vi "编辑Limit_Line.vi"(9 "引用":refnum<vi>, 11 "Data In":string[](array[string])) -> (1 "Operate":string, 2 "OK？":bool, 3 "Data Out":string[](array[string]))   [LabVIEW 2020]
panel:
  out "Unit 5":string
  out "Unit 4":string
  in  "End Response":dbl
  out "Unit 3":string="Hz"
  in  "End Stimulus":dbl format="%#.0f"
  out "Unit 2":string="Hz"
  in  "复制":bool
  in  "删除":bool
  in  "取消":bool
  in  "确定":bool
  in  "Begin Response":dbl
  in  "Type":u16(ring) items=["OFF", "MAX", "MIN"]
  in  "Begin Stimulus":dbl format="%#.0f"
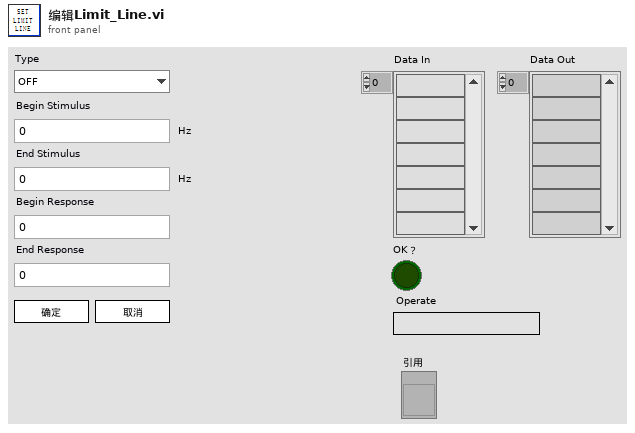
[diagram p1: front panel]
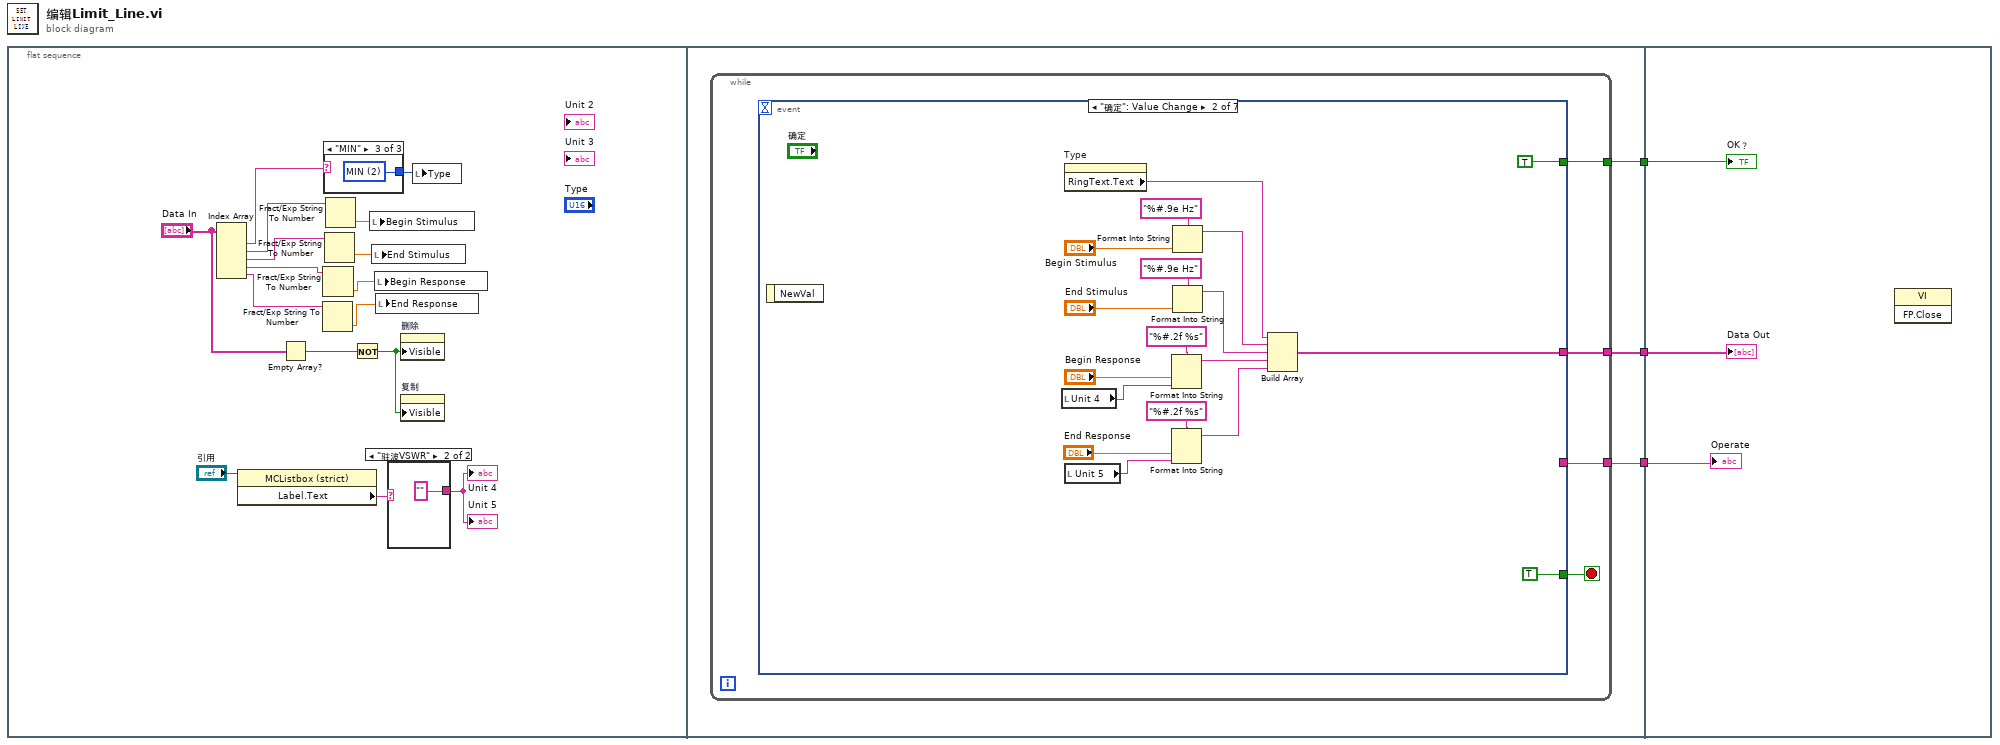
[diagram p0: block diagram]
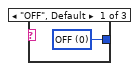
[diagram p2: hidden frame]
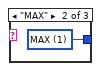
[diagram p3: hidden frame]
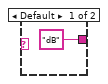
[diagram p4: hidden frame]
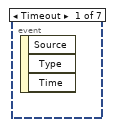
[diagram p5: hidden frame]
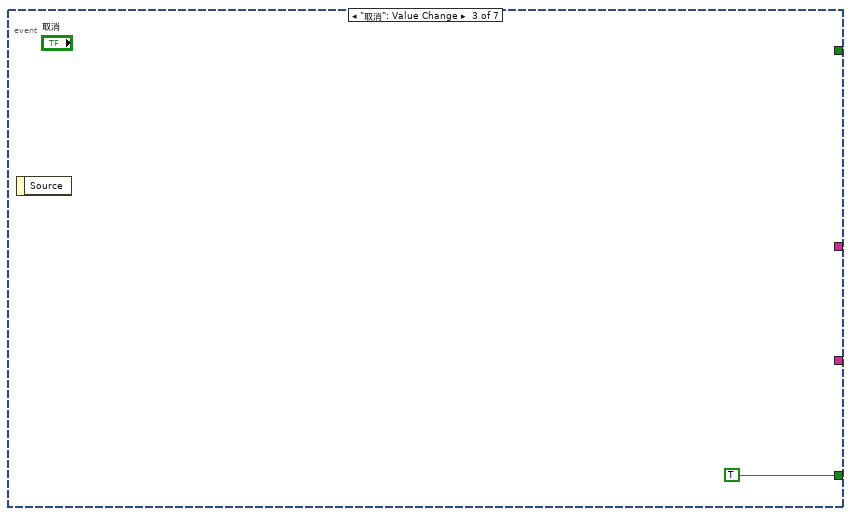
[diagram p6: hidden frame]
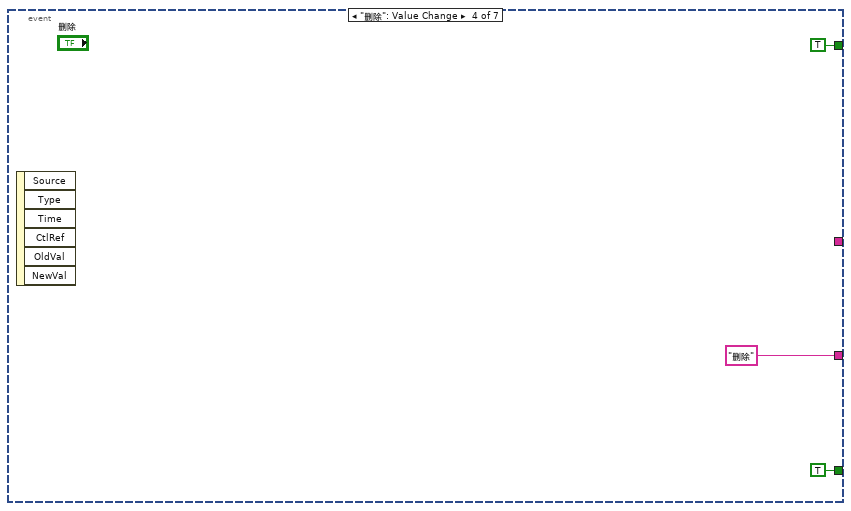
[diagram p7: hidden frame]
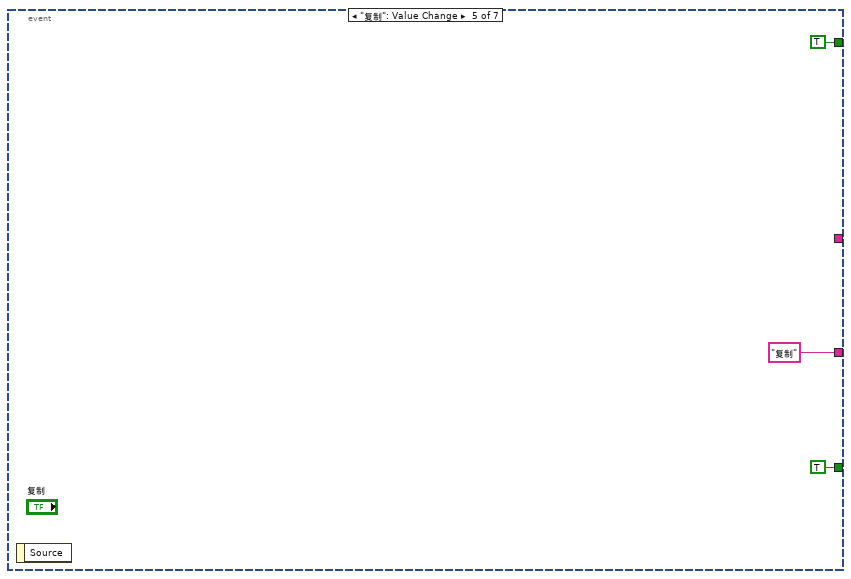
[diagram p8: hidden frame]
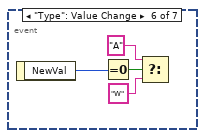
[diagram p9: hidden frame]
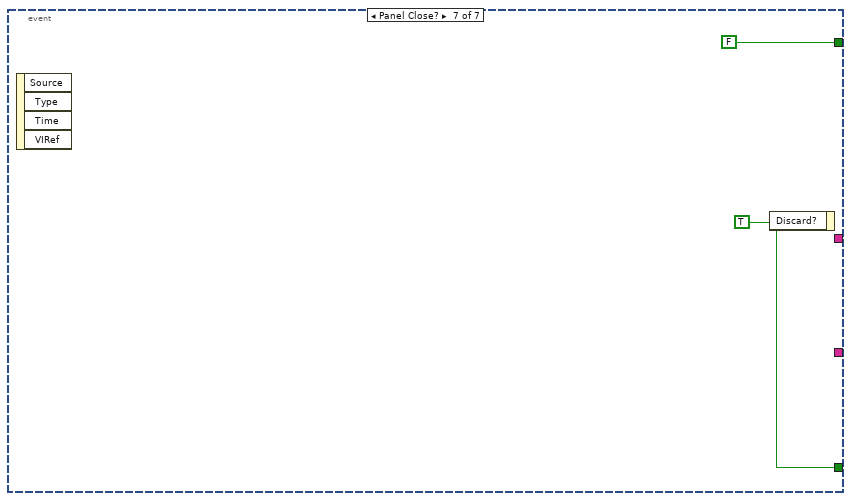
[diagram p10: hidden frame]
diagram:
  n1 = flat-sequence {
    tunnel: [w27] -> w3
    tunnel: [w26] -> w2
    tunnel: [w25] -> w1
    tunnel: w3 -> [w65]
    tunnel: w2 -> [w64]
    tunnel: w1 -> [w63]
    frame #0 {
      n2 = Index Array(array="Data In") -> (element #1=w12:string, element #2=w10:string, element #3=w8:string, element #4=w7:string, element #5=w5:string)  [unwired: 5 in]
      n3 = property class="MCListbox (strict)"(reference="引用") -> ("Label.Text"=w14:string)  [unwired: 1 in, 2 out]
      n4 = Empty Array?(array="Data In") -> (empty?=w17:bool)
      n5 = Fract/Exp String To Number(string=w5) -> (number=w4:dbl)  [unwired: 3 in, 1 out]
      n6 = Fract/Exp String To Number(string=w7) -> (number=w6:dbl)  [unwired: 3 in, 1 out]
      n7 = case shown="\"MIN\"" w12 {
        tunnel: [w20 w21 w22] -> w11
        frame "OFF", Default {
          w20 = u16 0 items=["OFF", "MAX", "MIN"] ("Type")
        }
        frame "MAX" {
          w21 = u16 1 items=["OFF", "MAX", "MIN"] ("Type")
        }
        frame "MIN" {
          w22 = u16 2 items=["OFF", "MAX", "MIN"] ("Type")
        }
      }
      n8 = Fract/Exp String To Number(string=w8) -> (number=w19:dbl)  [unwired: 3 in, 1 out]
      n9 = Fract/Exp String To Number(string=w10) -> (number=w9:dbl)  [unwired: 3 in, 1 out]
      n10 = Not(x=w17) -> (.not. x?=w16:bool)
      n11 = local write "Begin Stimulus"(w9) -> ()
      n12 = local write "End Stimulus"(w19) -> ()
      n13 = local write "Begin Response"(w6) -> ()
      n14 = local write "End Response"(w4) -> ()
      n15 = case shown="\"驻波VSWR\"" w14 {
        tunnel: ["dB" ""] -> w15
        frame Default {
        }
        frame "驻波VSWR" {
        }
      }
      "Unit 4" <- w15
      "Unit 5" <- w15
      n16 = property on="删除" class="Bool"("Visible"=w16) -> ()  [unwired: 2 in, 2 out]
      n17 = property on="复制" class="Bool"("Visible"=w16) -> ()  [unwired: 2 in, 2 out]
      n18 = local write "Type"(w11) -> ()
    }
    frame #1 {
      n19 = while {
        tunnel: [w30] -> w27
        tunnel: [w29] -> w26
        tunnel: [w28] -> w25
        stop <- w31 stop-if-true
        n20 = event shown="[1] \"确定\": Value Change" {
          selector: _ -> [_ _ _ _ _ _ _]
          dyn-events: _ -> [_ _ _ _ _ _ _]
          timeout: _ -> [_ _ _ _ _ _ _]
          tunnel: [_ TRUE ("放弃？") TRUE ("放弃？") TRUE ("放弃？") TRUE ("放弃？") _ w62] -> w31
          tunnel: [_ TRUE ("OK？") _ TRUE ("OK？") TRUE ("OK？") _ FALSE ("OK？")] -> w30
          tunnel: [_ w42 _ _ _ _ _] -> w29
          tunnel: [_ _ _ "删除" "复制" _ _] -> w28
          event Timeout {
            n21 = event-data() -> ()  [unwired: 1 in, 3 out]
          }
          event "确定": Value Change {
            n22 = event-data() -> ()  [unwired: 1 in, 1 out]
            n23 = local read "Unit 4"() -> (w33:string)
            n24 = property on="Type" class="Ring (strict)"() -> ("RingText.Text"=w41:string)  [unwired: 2 in, 2 out]
            n25 = local read "Unit 5"() -> (w32:string)
            n26 = Format Into String(format string="%#.2f %s" ("格式字符串"), "Begin Response", w33) -> (resulting string=w34:string)  [unwired: 2 in, 1 out]
            n27 = Format Into String(format string="%#.2f %s" ("格式字符串"), "End Response", w32) -> (resulting string=w45:string)  [unwired: 2 in, 1 out]
            n28 = Format Into String(format string="%#.9e Hz" ("格式字符串"), "Begin Stimulus") -> (resulting string=w46:string)  [unwired: 2 in, 1 out]
            n29 = Format Into String(format string="%#.9e Hz" ("格式字符串"), "End Stimulus") -> (resulting string=w38:string)  [unwired: 2 in, 1 out]
            n30 = Build Array(w41, w46, w38, w34, w45) -> (w42:string[])
          }
          event "取消": Value Change {
            n31 = event-data() -> ()  [unwired: 1 in, 1 out]
          }
          event "删除": Value Change {
            n32 = event-data() -> ()  [unwired: 1 in, 6 out]
          }
          event "复制": Value Change {
            n33 = event-data() -> ()  [unwired: 1 in, 1 out]
          }
          event "Type": Value Change {
            n34 = event-data() -> ("NewVal"=w60:u16)  [unwired: 1 in]
            n35 = Equal To 0?(x=w60) -> (x = 0?=w59:bool)
            n36 = Select(t="A", s=w59, f="W") -> ()  [unwired: 1 out]
          }
          event Panel Close? {
            w62 = TRUE ("放弃？")
            n37 = event-data() -> ()  [unwired: 1 in, 4 out]
            n38 = event-data("Discard?"=w62) -> ()  [unwired: 1 in, 1 out]
          }
        }
      }
    }
    frame #2 {
      n39 = invoke class="VI" method="FP.Close"() -> ()  [unwired: 3 in, 3 out]
      "OK？" <- w65
      "Data Out" <- w64
      "Operate" <- w63
    }
  }
